vi "Final Project Read File.vi"() -> ()   [LabVIEW 2017]
panel:
  out "Random Number      User Guess":dbl[][](array[numeric])
  # "Jay Patel\nDr. Kaputa\nBME 3120\n26 April 2018\n\nThis VI lets the user read the data collected from the guessing game."
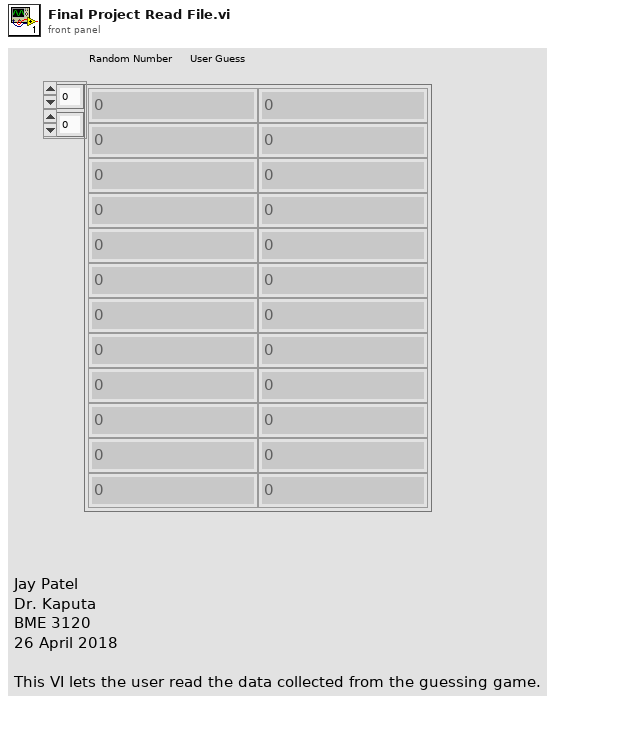
[diagram p1: front panel]
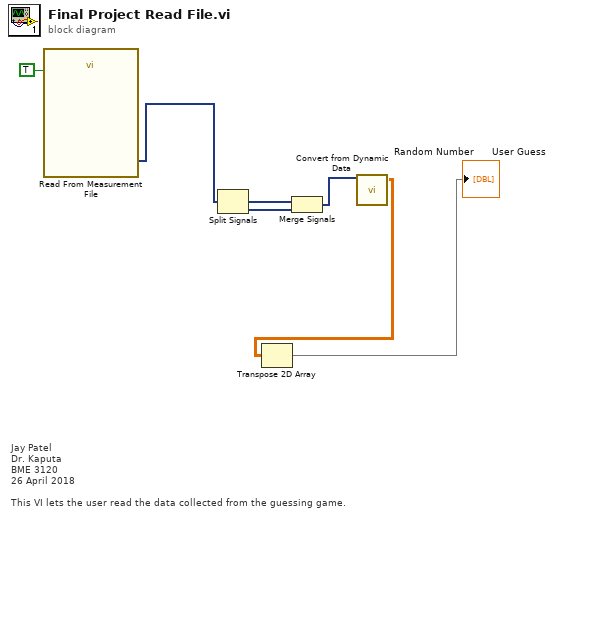
[diagram p0: block diagram]
diagram:
  # "Jay Patel\nDr. Kaputa\nBME 3120\n26 April 2018\n\nThis VI lets the user read the data collected from the guessing game."
  n1 = call "Read From Measurement File"("Enable"=TRUE) -> ("Signals"=w3:dynamicdata)  [unwired: 5 in, 5 out]
  n2 = Split Signals(w3) -> (w6:dynamicdata, w5:dynamicdata)  [unwired: 3 in, 1 out]
  n3 = Merge Signals(w6, w5) -> (w4:dynamicdata)
  n4 = call "Convert from Dynamic Data"("Dynamic Data Type"=w4) -> ("Array"=w2:dbl[][])  [unwired: 3 in]
  n5 = Transpose 2D Array(2D array=w2) -> (transposed array=→"Random Number      User Guess":dbl[][])
